vi "GetObjectInfo.vi"(9 "path":string, 10 "Ftp":refnum<k24>, 11 "error in":errorcluster) -> (1 "Info":T1, 3 "error out":errorcluster)   [LabVIEW 2023, in "UnderAutomation.Fanuc.lvlib"]
uses:
  UnderAutomation.Fanuc.lvlib
  C:/Users/fg/Documents/Fanuc.vi/LabVIEW_2024/UnderAutomation.Fanuc/lib/UnderAutomation.Fanuc.dll
  LabVIEW_2024/UnderAutomation.Fanuc/lib/UnderAutomation.Fanuc.dll
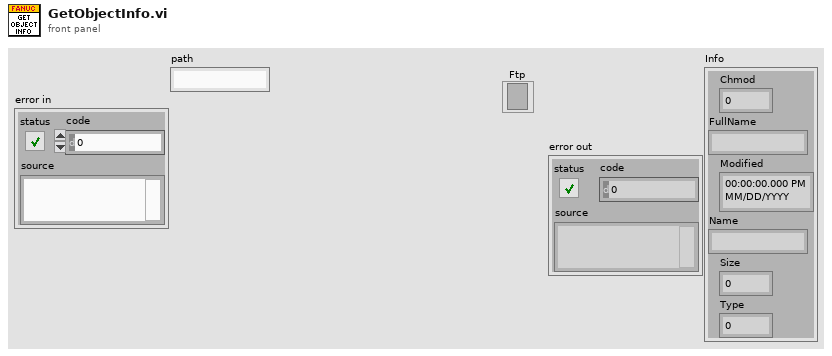
[diagram p1: front panel]
types:
  T1 = cluster{"Chmod":i32, "FullName":string, "Modified":timestamp, "Name":string, "Size":i64, "Type":i32}
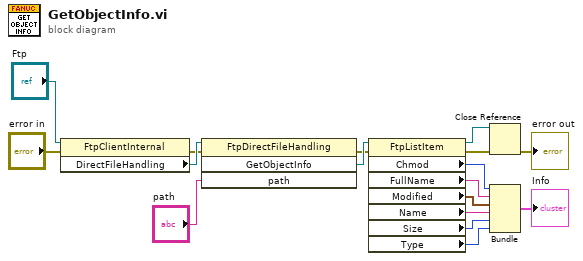
[diagram p0: block diagram]
diagram:
  n1 = property class="FtpClientInternal"(reference="Ftp", error in="error in") -> (error out=w13:errorcluster, "DirectFileHandling"=w15:refnum<k24>)  [unwired: 1 out]
  n2 = invoke class="FtpDirectFileHandling" method="GetObjectInfo"(reference=w15, error in=w13, "path"="path") -> (error out=w3:errorcluster, "GetObjectInfo"=w12:refnum<k24>)  [unwired: 1 in, 2 out]
  n3 = property class="FtpListItem"(reference=w12, error in=w3) -> (reference out=w1:refnum<k24>, error out=w2:errorcluster, "Chmod"=w11:i32, "FullName"=w10:string, "Modified"=w9:timestamp, "Name"=w8:string, "Size"=w7:i64, "Type"=w6:i32)
  n4 = Close Reference(reference=w1, error in (no error)=w2) -> (error out=→"error out":errorcluster)
  n5 = Bundle("Chmod"=w11, "FullName"=w10, "Modified"=w9, "Name"=w8, "Size"=w7, "Type"=w6) -> (→"Info":T1)  [unwired: 1 in]
